vi "startTestSeries.vi"(0 "EnabledState in":refnum<class "EnabledState.lvclass">, 1 "Model in":refnum<class "Model.lvclass">, 2 "Serial Number":string, 3 "Operator":string, 4 "Comments":string, 5 "error in (no error)":errorcluster) -> (14 "EnabledState out":refnum<class "EnabledState.lvclass">, 15 "Model out":refnum<class "Model.lvclass">, 19 "error out":errorcluster)   [LabVIEW 2015, in "EnabledState.lvclass"]
uses:
  EnabledState.lvclass
  Model/Model/Model.lvclass
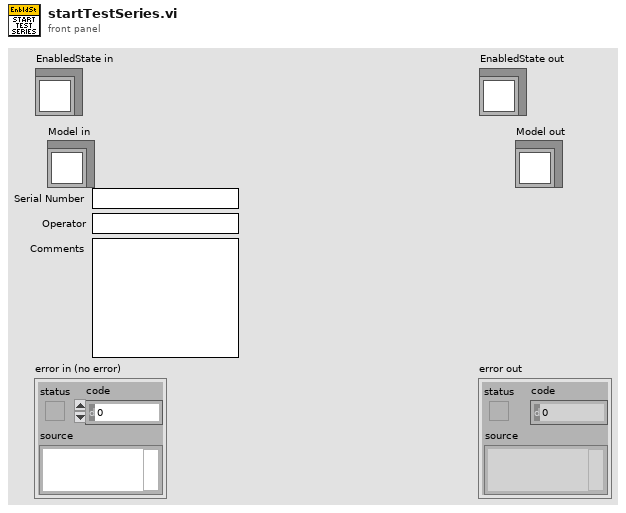
[diagram p1: front panel]
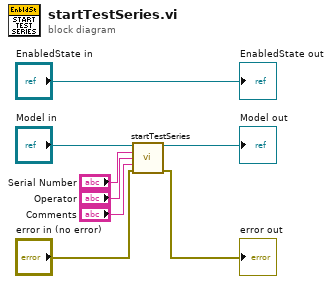
[diagram p0: block diagram]
diagram:
  n1 = call "startTestSeries.vi"("Model in"="Model in", "Serial Number"="Serial Number", "Operator"="Operator", "Comments"="Comments", "error in (no error)"="error in (no error)") -> ("Model out"=→"Model out":refnum<class "Model.lvclass">, "error out"=→"error out":errorcluster)  [unwired: 9 in]
  "EnabledState out" <- "EnabledState in"
